vi "_Validate Mass Ranges.vi"(1 "error in":errorcluster, 2 "Expt#":i32, 3 "Mass Range":T1[](array[typedef]) {"Resolution Type" items=["High/High", "Medium/Medium", "Low/Low", "High/Medium", "High/Low", "Medium/High", "Medium/Low", "Low/High", "Low/Medium"]}) -> (0 "error out":errorcluster)   [LabVIEW 2015]
uses:
  Type/_RT Mass Range.ctl
  Type/_RT Res Type.ctl
  Type/_RT Active Ch.ctl
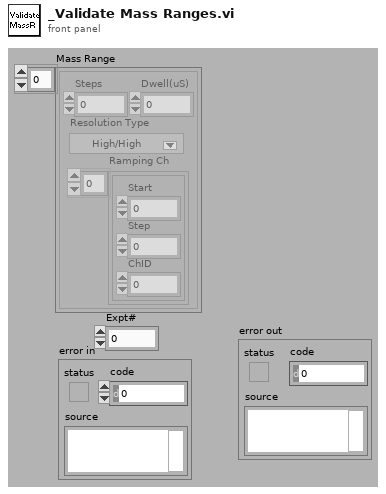
[diagram p1: front panel]
types:
  T1 = typedef "_RT Mass Range.ctl" = cluster{"Steps":i32, "Dwell(uS)":i32, "Resolution Type":T2, "Ramping Ch":T3[]}
  T2 = typedef "_RT Res Type.ctl" = u16
  T3 = typedef "_RT Active Ch.ctl" = cluster{"Start":i32, "Step":i32, "ChID":i32}
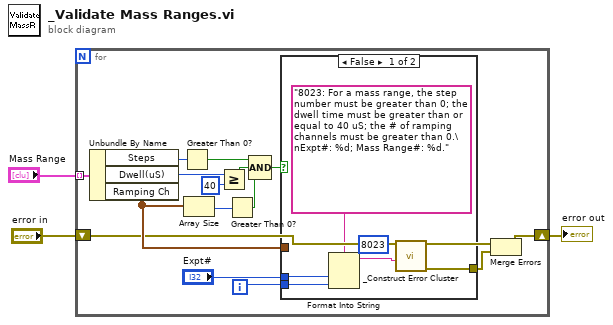
[diagram p0: block diagram]
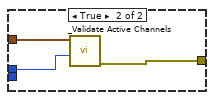
[diagram p2: hidden frame]
diagram:
  n1 = for {
    tunnel: "Mass Range" -> [w18] mode=indexing
    shift-right: [w6] -> w1
    shift-left: "error in" -> [w8]
    i -> [w4]
    n2 = Unbundle By Name(w18) -> ("Steps"=w17:i32, "Dwell(uS)"=w16:i32, "Ramping Ch"=w9:T3[])
    n3 = Greater Than 0?(x=w17) -> (x > 0?=w13:bool)
    n4 = Array Size(array=w9) -> (size(s)=w14:i32)
    n5 = Greater Or Equal?(x=w16, y=40) -> (x >= y?=w12:bool)
    n6 = Greater Than 0?(x=w14) -> (x > 0?=w11:bool)
    n7 = Compound Arithmetic op=AND(w13, w12, w11) -> (w10:bool)
    n8 = case shown="False" w10 {
      tunnel: w9 -> [_ w27]
      tunnel: [w24 w26] -> w7
      tunnel: "Expt#" -> [w23 w25]
      tunnel: w4 -> [w22 _]
      frame False {
        n9 = Format Into String(format string="8023: For a mass range, the step number must be greater than 0; the dwell time must be greater than or equal to 40 uS; the # of ramping channels must be greater than 0.\nExpt#: %d; Mass Range#: %d.", w23, w22) -> (resulting string=w20:string)  [unwired: 2 in, 1 out]
        n10 = call "_Construct Error Cluster.vi"("reason"=w20, "errorCode"=8023) -> ("error out"=w24:errorcluster)  [unwired: 2 in, 3 out]
      }
      frame True {
        n11 = call "_Validate Active Channels.vi"("Expt#"=w25, "Active Ch"=w27) -> ("error out"=w26:errorcluster)  [unwired: 4 in, 3 out]
      }
    }
    n12 = Merge Errors(w8, w7) -> (w6:errorcluster)
  }
  "error out" <- w1
